vi "Tower_Crane_Balance_Monitor_beta.vi"() -> ()   [LabVIEW 2018]
uses:
  <vilib>/vision/driver/IMAQdx.llb/IMAQdx Acquisition Mode.ctl
  <vilib>/userdefined/High Color/IMAQdx.ctl
  <vilib>/Utility/error.llb/DialogType.ctl
  <vilib>/vision/driver/NI_Vision_Acquisition_Software.lvlib
panel:
  in  "File Path":path
  out "error out 2":errorcluster
  in  "error in":errorcluster
  in  "停止 3":bool
  out "视频监控画面1":T1(plugin-control)
  out "new picture 4":picture caption="Opertion_Guide"
  out "new picture 3":picture caption="Opertion_Guide"
  out "new picture 2":picture caption="Opertion_Guide"
  out "stanard_section 2":picture caption="配平状态"
  out "X倾斜角度 2":dbl caption="塔身X倾斜角度" format="%#_3g"
  out "Y倾斜角度  2":dbl caption="塔身Y倾斜角度" format="%#_3g"
  out "y轴倾角 2":dbl(knob) scale=0.0..5.0
  out "x轴倾角 2":dbl(knob) scale=0.0..5.0
  out "配平指示1":bool
  out "超声波雷达4":dbl format="%.3f"
  out "超声波雷达4 6":dbl(knob) scale=0.0..10.0
  out "超声波雷达35":dbl format="%.3f"
  out "?":dbl(knob) scale=0.0..10.0
  out "超声波雷达2":dbl format="%.3f"
  out "超声波雷达2":dbl(knob) scale=0.0..10.0
  out "超声波雷达1":dbl format="%.3f"
  out "超声波雷达1":dbl(knob) scale=0.0..10.0
  out "起升高度（m）":dbl caption="起升高度（cm）" format="%#_3g"
  out "变幅长度（m）":dbl format="%#_3g"
  out "风速（m/s）":dbl format="%.3f"
  out "Y倾斜角度":dbl caption="套架Y倾斜角度" format="%#_3g"
  out "X倾斜角度":dbl caption="套架X倾斜角度" format="%#_3g"
  out "回转角度（°）":dbl format="%#_3g"
  out "回转角度":dbl(knob) scale=0.0..10.0
  out "风速":dbl(knob) scale=0.0..10.0
  out "变幅长度":dbl(knob) scale=0.0..140.0
  out "y轴倾角":dbl(knob) scale=0.0..5.0
  out "x轴倾角":dbl(knob) scale=0.0..5.0
  out "起升高度":dbl(slide) caption="顶升高度          (cm)" scale=0.0..180.0
  out "section_connect":picture caption="引进节连接"
  out "rotary_support":picture caption="下回转支座"
  out "stanard_section":picture caption="引进节"
  out "pin_shaft":picture caption="爬爪"
  out "jacking_beam":picture caption="顶升横梁"
  out "new picture":picture caption="Opertion_Guide"
  out "引进滑轮":bool
  out "引进节螺栓4":bool
  out "引进节螺栓3":bool
  out "引进节螺栓2":bool
  out "引进节螺栓1":bool
  out "下回转螺栓4":bool
  out "下回转螺栓3":bool
  out "下回转螺栓2":bool
  out "下回转螺栓1":bool
  out "爬爪右侧":bool
  out "爬爪左侧":bool
  out "横梁右侧":bool
  out "横梁左侧":bool
  in  "倾角串口号 2":refnum<visa-resource-name>
  in  "开始配平":bool
  in  "倾角串口号":refnum<visa-resource-name>
  in  "风速串口号":refnum<visa-resource-name>
  in  "回转编码器":refnum<visa-resource-name>
  in  "变幅编码器":refnum<visa-resource-name>
  in  "高度编码器":refnum<visa-resource-name>
  in  "顶升开关":bool
  in  "滚轮直径D":dbl
  out "倾角读取缓冲区 2":string caption="倾角读取缓冲区"
  out "子字符串 4":string
  out "子字符串 3":string
  out "子字符串 2":string
  out "子字符串":string
  out "数据输出 2":string
  out "esp32的IP地址 2":string
  out "信息来源的端口 2":u16
  in  "清空 2":bool
  out "esp32的IP地址":string
  out "回转圈数":dbl
  out "回转编码器读取缓冲区":string
  out "回转单圈值":dbl
  out "回转编码器错误输出":string
  out "变幅圈数":dbl
  out "小车蝙蝠编码器读取缓冲区":string
  out "变幅单圈值":dbl
  out "回转编码器错误输出1":string
  out "倾角读取缓冲区":string
  out "Wind_Speed_Data":string
  out "风速传感器错误输出":string
  out "操作规范":string
  out "起升圈数":dbl
  out "起升高度编码器读取缓冲区 2":string
  out "起升单圈值":dbl
  out "起升高度编码器数值":dbl
  out "高度编码器错误输出1":string
  out "data out":string
  out "数据输出":string
  out "信息来源的端口":u16
  in  "停止":bool
  in  "清空":bool
types:
  T1 = typedef "IMAQ Image.ctl" = refnum<image>
  T2 = typedef "IMAQdx.ctl" = refnum<k21>
  T3 = typedef "NI_Vision_Acquisition_Software.lvlib/IMAQdx Acquisition Mode.ctl" = enum32{"One Shot", "Continuous"}
  T4 = typedef "DialogType.ctl" = u16
  T5 = typedef "imagedata.ctl" = cluster{"image type":i32, "image depth":i32, "image":u8[], "mask":u8[], "colors":u32[], "Rectangle":cluster{"left":i16, "top":i16, "right":i16, "bottom":i16}}
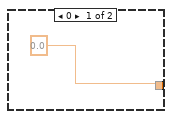
[diagram p2: hidden frame]
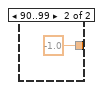
[diagram p4: hidden frame]
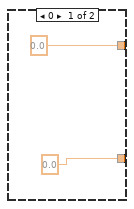
[diagram p9: hidden frame]
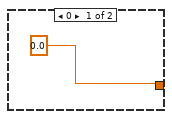
[diagram p14: hidden frame]
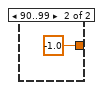
[diagram p16: hidden frame]
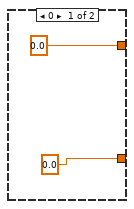
[diagram p17: hidden frame]
diagram:
  n1 = UDP Open(11:u16 8081 ("端口")) -> (port=w33:refnum<k16>, 0:w31:errorcluster)  [unwired: 4 in, 1 out]
  n2 = UDP Open(11:u16 8080 ("端口")) -> (port=w39:refnum<k16>, 0:w38:errorcluster)  [unwired: 4 in, 1 out]
  n3 = UDP Open(11:u16 8082 ("端口")) -> (port=w27:refnum<k16>, 0:w28:errorcluster)  [unwired: 4 in, 1 out]
  n4 = while {
    tunnel: w39 -> [w113]
    tunnel: w38 -> [w108]
    tunnel: [w141] -> w37
    tunnel: [w138] -> w36
    tunnel: w33 -> [w103]
    tunnel: [w101] -> w32
    tunnel: w31 -> [w99]
    tunnel: [w90] -> w30
    tunnel: w28 -> [w82]
    tunnel: w27 -> [w86]
    tunnel: [w81] -> w26
    tunnel: [w80] -> w25
    stop <- "停止" stop-if-true
    n5 = String To IP(1:"192.168.16.233" ("名称")) -> (0:w96:u32)
    n6 = String To IP(1:"192.168.16.236" ("名称")) -> (0:w110:u32)
    n7 = String To IP(1:"192.168.16.107" ("名称")) -> (0:w85:u32)
    n8 = UDP Write(address=w96, port or service name=u16 7780 ("端口或服务名称"), connection ID=w103, 8:w99) -> (error out=w100:errorcluster, 3:w102:refnum<k16>)  [unwired: 2 in]
    n9 = UDP Write(address=w110, port or service name=u16 7788 ("端口或服务名称"), connection ID=w113, 8:w108) -> (error out=w109:errorcluster, 3:w112:refnum<k16>)  [unwired: 2 in]
    n10 = Unbundle By Name(w82) -> ("code"=w83:i32)
    n11 = case shown="60" w83 {
      frame 0, Default {
      }
      frame 60 {
        n12 = Wait (ms)(milliseconds to wait=u32 5000 ("等待时间（毫秒）")) -> ()  [unwired: 1 out]
        n13 = One Button Dialog(message="目标端口被占用" ("消息"), button name ("OK")="难受" ("按钮名称（“确定”）")) -> ()  [unwired: 1 out]
      }
    }
    n14 = disable-structure shown="禁用" {
      disable-tunnel: [w142 _] -> w65
      frame Disabled {
        n15 = case shown="1, 默认" 1 {
          tunnel: [0.0 w150] -> w142
          frame 0 {
          }
          frame 1, Default {
            w148 = T4 0 items=["无对话框", "确定信息", "继续或停止信息", "确定信息＋警告", "继续/停止+警告"] ("type of dialog (OK msg:1)")
            w151 = i32[] [1, 3, 0, 2, 0, 2, 101, 203]  # 读指令
            n16 = Byte Array To String(unsigned byte array=w151) -> (string=w168:string)
            n17 = flat-sequence {
              tunnel: "变幅编码器" -> [w196]
              tunnel: [w196] -> w145
              frame #0 {
                n18 = Wait (ms)(milliseconds to wait=5) -> ()  [unwired: 1 out]
              }
            }
            n19 = flat-sequence {
              tunnel: [w194] -> w167
              tunnel: w168 -> [w194]
              frame #0 {
                n20 = Wait (ms)(milliseconds to wait=5) -> ()  [unwired: 1 out]
              }
            }
            n21 = VISA Write(VISA resource name=w145, write buffer=w167) -> (VISA resource name out=w159:refnum<visa-resource-name>)  [unwired: 1 in, 2 out]
            n22 = flat-sequence {
              tunnel: [w192] -> w160
              tunnel: w159 -> [w192]
              frame #0 {
                n23 = Wait (ms)(milliseconds to wait=5) -> ()  [unwired: 1 out]
              }
            }
            n24 = VISA Read(VISA resource name=w160, byte count=u32 9 ("字节总数")) -> (VISA resource name out=w176:refnum<visa-resource-name>, read buffer=w166:string, error out=w147:errorcluster)  [unwired: 1 in, 1 out]
            "小车蝙蝠编码器读取缓冲区" <- w166
            n25 = call <vilib>:"Simple Error Handler.vi"("type of dialog (OK msg:1)"=w148, "error in (no error)"=w147) -> ("error?"=w149:bool)  [unwired: 3 in, 4 out]
            n26 = case shown="真" w149 {
              frame False {
              }
              frame True {
                "回转编码器错误输出1" <- "小车变幅编码器丢失信号" ("九轴错误输出1")
              }
            }
            n27 = String To Byte Array(string=w166) -> (unsigned byte array=w174:u8[])
            n28 = VISA Flush I/O Buffer(VISA resource name=w176, mask (16)=64) -> (VISA resource name out=w175:refnum<visa-resource-name>)  [unwired: 1 in, 1 out]
            n29 = Index Array ("索引数组")(array=w174, index=3) -> (element=w161:u8)
            n30 = Index Array(array=w174, index=4) -> (element=w165:u8)
            n31 = Index Array ("索引数组")(array=w174, index=5) -> (element=w169:u8)
            n32 = Index Array(array=w174, index=6) -> (element=w173:u8)
            n33 = VISA Flush I/O Buffer(VISA resource name=w175, mask (16)=128) -> ()  [unwired: 1 in, 2 out]
            n34 = Number To Hexadecimal String(2:w161) -> (0:w164:string)  [unwired: 1 in]
            n35 = Number To Hexadecimal String(2:w165) -> (0:w163:string)  [unwired: 1 in]
            n36 = Number To Hexadecimal String(2:w169) -> (0:w172:string)  [unwired: 1 in]
            n37 = Number To Hexadecimal String(2:w173) -> (0:w171:string)  [unwired: 1 in]
            n38 = Concatenate Strings(w164, w163) -> (w162:string)
            n39 = Concatenate Strings(w172, w171) -> (w170:string)
            n40 = Hexadecimal String To Number(string=w162) -> (number=w177:u32)  [unwired: 2 in, 1 out]
            "变幅圈数" <- w177
            n41 = Hexadecimal String To Number(string=w170) -> (number=w178:u32)  [unwired: 2 in, 1 out]
            "变幅单圈值" <- w178
            n42 = case shown="默认" w177 {
              selector: w177 -> [w184 _]
              tunnel: w178 -> [w183 _]
              tunnel: [w182 -1.0] -> w150
              frame Default {
                n43 = Multiply(x=w184, y=1024.0) -> (x*y=w189:dbl)
                n44 = Add(x=w189, y=w183) -> (x+y=w190:dbl)
                n45 = Multiply(x=w190, y=0.001) -> (x*y=w187:dbl)
                n46 = Multiply(x=w187, y=3.141592653589793) -> (x*y=w188:dbl)
                n47 = Multiply(x=w188, y=3.0) -> (x*y=w182:dbl)
              }
              frame 90..99 {
              }
            }
          }
        }
      }
      frame Enabled {
      }
    }
    "变幅长度（m）" <- w65
    "变幅长度" <- w65
    n48 = Unbundle By Name(w108) -> ("code"=w132:i32)
    n49 = Unbundle By Name(w99) -> ("code"=w98:i32)
    n50 = case shown="60" w132 {
      frame 0, Default {
      }
      frame 60 {
        n51 = Wait (ms)(milliseconds to wait=u32 5000 ("等待时间（毫秒）")) -> ()  [unwired: 1 out]
        n52 = One Button Dialog(message="目标端口被占用" ("消息"), button name ("OK")="难受" ("按钮名称（“确定”）")) -> ()  [unwired: 1 out]
      }
    }
    n53 = case shown="60" w98 {
      frame 0, Default {
      }
      frame 60 {
        n54 = Wait (ms)(milliseconds to wait=u32 5000 ("等待时间（毫秒）")) -> ()  [unwired: 1 out]
        n55 = One Button Dialog(message="目标端口被占用" ("消息"), button name ("OK")="难受" ("按钮名称（“确定”）")) -> ()  [unwired: 1 out]
      }
    }
    n56 = case shown="1, 默认" 1 {
      tunnel: [0.0 w264] -> w64
      frame 0 {
      }
      frame 1, Default {
        w262 = T4 0 items=["无对话框", "确定信息", "继续或停止信息", "确定信息＋警告", "继续/停止+警告"] ("type of dialog (OK msg:1)")
        w265 = i32[] [1, 3, 0, 2, 0, 2, 101, 203]  # 读指令
        n57 = Byte Array To String(unsigned byte array=w265) -> (string=w282:string)
        n58 = flat-sequence {
          tunnel: "回转编码器" -> [w312]
          tunnel: [w312] -> w259
          frame #0 {
            n59 = Wait (ms)(milliseconds to wait=5) -> ()  [unwired: 1 out]
          }
        }
        n60 = flat-sequence {
          tunnel: [w310] -> w281
          tunnel: w282 -> [w310]
          frame #0 {
            n61 = Wait (ms)(milliseconds to wait=5) -> ()  [unwired: 1 out]
          }
        }
        n62 = VISA Write(VISA resource name=w259, write buffer=w281) -> (VISA resource name out=w273:refnum<visa-resource-name>)  [unwired: 1 in, 2 out]
        n63 = flat-sequence {
          tunnel: [w308] -> w274
          tunnel: w273 -> [w308]
          frame #0 {
            n64 = Wait (ms)(milliseconds to wait=5) -> ()  [unwired: 1 out]
          }
        }
        n65 = VISA Read(VISA resource name=w274, byte count=u32 9 ("字节总数")) -> (VISA resource name out=w290:refnum<visa-resource-name>, read buffer=w280:string, error out=w261:errorcluster)  [unwired: 1 in, 1 out]
        "回转编码器读取缓冲区" <- w280
        n66 = call <vilib>:"Simple Error Handler.vi"("type of dialog (OK msg:1)"=w262, "error in (no error)"=w261) -> ("error?"=w263:bool)  [unwired: 3 in, 4 out]
        n67 = case shown="真" w263 {
          frame False {
          }
          frame True {
            "回转编码器错误输出" <- "回转编码器丢失信号" ("九轴错误输出1")
          }
        }
        n68 = String To Byte Array(string=w280) -> (unsigned byte array=w288:u8[])
        n69 = VISA Flush I/O Buffer(VISA resource name=w290, mask (16)=64) -> (VISA resource name out=w289:refnum<visa-resource-name>)  [unwired: 1 in, 1 out]
        n70 = Index Array ("索引数组")(array=w288, index=3) -> (element=w275:u8)
        n71 = Index Array(array=w288, index=4) -> (element=w279:u8)
        n72 = Index Array ("索引数组")(array=w288, index=5) -> (element=w283:u8)
        n73 = Index Array(array=w288, index=6) -> (element=w287:u8)
        n74 = VISA Flush I/O Buffer(VISA resource name=w289, mask (16)=128) -> ()  [unwired: 1 in, 2 out]
        n75 = Number To Hexadecimal String(2:w275) -> (0:w278:string)  [unwired: 1 in]
        n76 = Number To Hexadecimal String(2:w279) -> (0:w277:string)  [unwired: 1 in]
        n77 = Number To Hexadecimal String(2:w283) -> (0:w286:string)  [unwired: 1 in]
        n78 = Number To Hexadecimal String(2:w287) -> (0:w285:string)  [unwired: 1 in]
        n79 = Concatenate Strings(w278, w277) -> (w276:string)
        n80 = Concatenate Strings(w286, w285) -> (w284:string)
        n81 = Hexadecimal String To Number(string=w276) -> (number=w291:u32)  [unwired: 2 in, 1 out]
        "回转圈数" <- w291
        n82 = Hexadecimal String To Number(string=w284) -> (number=w292:u32)  [unwired: 2 in, 1 out]
        "回转单圈值" <- w292
        n83 = case shown="默认" w291 {
          selector: w291 -> [w304 _]
          tunnel: w292 -> [w303 _]
          tunnel: [w295 -1.0] -> w264
          frame Default {
            n84 = Multiply(x=w304, y=1024.0) -> (x*y=w306:dbl)
            n85 = Add(x=w306, y=w303) -> (x+y=w302:dbl)
            n86 = Quotient & Remainder(x=w302, y=1024.0) -> (x-y*floor(x/y)=w297:dbl)  [unwired: 1 out]
            n87 = Divide(x=w297, y=1024.0) -> (x/y=w299:dbl)
            n88 = Multiply(x=w299, y=360.0) -> (x*y=w296:dbl)
            n89 = Divide(x=w296, y=10.0) -> (x/y=w295:dbl)
          }
          frame 90..99 {
          }
        }
      }
    }
    "回转角度（°）" <- w64
    "回转角度" <- w64
    n90 = disable-structure shown="禁用" {
      frame Disabled {
        n91 = case shown="1, 默认" 1 {
          tunnel: [0.0 w217] -> w211
          tunnel: [0.0 w223] -> w210
          frame 0 {
          }
          frame 1, Default {
            w220 = T4 0 items=["无对话框", "确定信息", "继续或停止信息", "确定信息＋警告", "继续/停止+警告"] ("type of dialog (OK msg:1)")
            w224 = i32[] [80, 3, 0, 61, 0, 3, 153, 134]  # 读指令
            # "javascript:placeObject(object906);"
            n92 = Byte Array To String(unsigned byte array=w224) -> (string=w236:string)
            n93 = flat-sequence {
              tunnel: "倾角串口号 2" -> [w256]
              tunnel: [w256] -> w218
              frame #0 {
                n94 = Wait (ms)(milliseconds to wait=5) -> ()  [unwired: 1 out]
              }
            }
            n95 = flat-sequence {
              tunnel: [w254] -> w215
              tunnel: w236 -> [w254]
              frame #0 {
                n96 = Wait (ms)(milliseconds to wait=5) -> ()  [unwired: 1 out]
              }
            }
            n97 = VISA Write(VISA resource name=w218, write buffer=w215) -> (VISA resource name out=w232:refnum<visa-resource-name>)  [unwired: 1 in, 2 out]
            n98 = flat-sequence {
              tunnel: w232 -> [w252]
              tunnel: [w252] -> w233
              frame #0 {
                n99 = Wait (ms)(milliseconds to wait=5) -> ()  [unwired: 1 out]
              }
            }
            n100 = VISA Read(VISA resource name=w233, byte count=u32 11 ("字节总数")) -> (VISA resource name out=w240:refnum<visa-resource-name>, read buffer=w216:string, error out=w221:errorcluster)  [unwired: 1 in, 1 out]
            "倾角读取缓冲区 2" <- w216
            n101 = call <vilib>:"Simple Error Handler.vi"("type of dialog (OK msg:1)"=w220, "error in (no error)"=w221) -> ("error?"=w222:bool)  [unwired: 3 in, 4 out]
            n102 = String To Byte Array(string=w216) -> (unsigned byte array=w241:u8[])
            n103 = VISA Flush I/O Buffer(VISA resource name=w240, mask (16)=64) -> (VISA resource name out=w239:refnum<visa-resource-name>)  [unwired: 1 in, 1 out]
            n104 = case shown="真" w222 {
              frame False {
              }
              frame True {
              }
            }
            n105 = Index Array(array=w241, index=5) -> (element=w238:u8)
            n106 = Index Array(array=w241, index=6) -> (element=w237:u8)
            n107 = Index Array(array=w241, index=3) -> (element=w235:u8)
            n108 = Index Array(array=w241, index=4) -> (element=w234:u8)
            n109 = formula code="z=((x<<8)|y)/32768*180;"("x"=w238, "y"=w237) -> ("z"=w243:dbl)
            n110 = formula code="z=((x<<8)|y)/32768*180;"("x"=w235, "y"=w234) -> ("z"=w242:dbl)
            n111 = VISA Flush I/O Buffer(VISA resource name=w239, mask (16)=128) -> ()  [unwired: 1 in, 2 out]
            n112 = case shown="300..360" w243 {
              tunnel: [w248 w250] -> w217
              tunnel: w243 -> [w248 w249]
              frame Default {
              }
              frame 300..360 {
                n113 = Subtract(x=360.0, y=w249) -> (x-y=w250:dbl)
              }
            }
            n114 = case shown="300..360" w242 {
              tunnel: [w244 w246] -> w223
              tunnel: w242 -> [w244 w245]
              frame Default {
              }
              frame 300..360 {
                n115 = Subtract(x=360.0, y=w245) -> (x-y=w246:dbl)
              }
            }
          }
        }
        "X倾斜角度 2" <- w210
        "Y倾斜角度  2" <- w211
        "y轴倾角 2" <- w211
        "x轴倾角 2" <- w210
        n116 = Number To Fractional String(number=w210) -> ()  [unwired: 3 in, 1 out]
        n117 = Number To Fractional String(number=w211) -> ()  [unwired: 3 in, 1 out]
      }
      frame Enabled {
      }
    }
    n118 = case shown="1, 默认" 1 {
      tunnel: [0.0 w400] -> w72
      frame 0 {
      }
      frame 1, Default {
        w398 = T4 0 items=["无对话框", "确定信息", "继续或停止信息", "确定信息＋警告", "继续/停止+警告"] ("type of dialog (OK msg:1)")
        w401 = i32[] [1, 3, 0, 2, 0, 2, 101, 203]  # 读指令
        n119 = Byte Array To String(unsigned byte array=w401) -> (string=w417:string)
        n120 = flat-sequence {
          tunnel: "高度编码器" -> [w446]
          tunnel: [w446] -> w395
          frame #0 {
            n121 = Wait (ms)(milliseconds to wait=5) -> ()  [unwired: 1 out]
          }
        }
        n122 = flat-sequence {
          tunnel: [w444] -> w416
          tunnel: w417 -> [w444]
          frame #0 {
            n123 = Wait (ms)(milliseconds to wait=5) -> ()  [unwired: 1 out]
          }
        }
        n124 = VISA Write(VISA resource name=w395, write buffer=w416) -> (VISA resource name out=w409:refnum<visa-resource-name>)  [unwired: 1 in, 2 out]
        n125 = flat-sequence {
          tunnel: [w442] -> w410
          tunnel: w409 -> [w442]
          frame #0 {
            n126 = Wait (ms)(milliseconds to wait=5) -> ()  [unwired: 1 out]
          }
        }
        n127 = VISA Read(VISA resource name=w410, byte count=u32 9 ("字节总数")) -> (VISA resource name out=w425:refnum<visa-resource-name>, read buffer=w426:string, error out=w397:errorcluster)  [unwired: 1 in, 1 out]
        "起升高度编码器读取缓冲区 2" <- w426
        n128 = call <vilib>:"Simple Error Handler.vi"("type of dialog (OK msg:1)"=w398, "error in (no error)"=w397) -> ("error?"=w399:bool)  [unwired: 3 in, 4 out]
        n129 = case shown="假" w399 {
          frame False {
          }
          frame True {
            "高度编码器错误输出1" <- "起升高度编码器丢失信号" ("九轴错误输出1")
          }
        }
        n130 = String To Byte Array(string=w426) -> (unsigned byte array=w423:u8[])
        n131 = VISA Flush I/O Buffer(VISA resource name=w425, mask (16)=64) -> (VISA resource name out=w424:refnum<visa-resource-name>)  [unwired: 1 in, 1 out]
        n132 = Index Array ("索引数组")(array=w423, index=3) -> (element=w411:u8)
        n133 = Index Array(array=w423, index=4) -> (element=w415:u8)
        n134 = Index Array ("索引数组")(array=w423, index=5) -> (element=w418:u8)
        n135 = Index Array(array=w423, index=6) -> (element=w422:u8)
        n136 = VISA Flush I/O Buffer(VISA resource name=w424, mask (16)=128) -> ()  [unwired: 1 in, 2 out]
        n137 = Number To Hexadecimal String(2:w411) -> (0:w414:string)  [unwired: 1 in]
        n138 = Number To Hexadecimal String(2:w415) -> (0:w413:string)  [unwired: 1 in]
        n139 = Number To Hexadecimal String(2:w418) -> (0:w421:string)  [unwired: 1 in]
        n140 = Number To Hexadecimal String(2:w422) -> (0:w420:string)  [unwired: 1 in]
        n141 = Concatenate Strings(w414, w413) -> (w412:string)
        n142 = Concatenate Strings(w421, w420) -> (w419:string)
        n143 = Hexadecimal String To Number(string=w412) -> (number=w427:u32)  [unwired: 2 in, 1 out]
        "起升圈数" <- w427
        n144 = Hexadecimal String To Number(string=w419) -> (number=w428:u32)  [unwired: 2 in, 1 out]
        "起升单圈值" <- w428
        n145 = case shown="默认" w427 {
          selector: w427 -> [w437 _]
          tunnel: w428 -> [w438 _]
          tunnel: [w430 -1.0] -> w400
          frame Default {
            n146 = Multiply(x=w437, y=1024.0) -> (x*y=w440:dbl)
            n147 = Add(x=w440, y=w438) -> (x+y=w436:dbl)
            "起升高度编码器数值" <- w436
            n148 = Divide(x=w436, y=1024.0) -> (x/y=w434:dbl)
            n149 = Multiply(x=w434, y=3.141592653589793) -> (x*y=w432:dbl)
            n150 = Multiply(x=w432, y="滚轮直径D") -> (x*y=w430:dbl)
          }
          frame 90..99 {
          }
        }
      }
    }
    "起升高度（m）" <- w72
    "起升高度" <- w72
    n151 = case shown="1, 默认" 1 {
      tunnel: [0.0 w322] -> w48
      tunnel: [0.0 w321] -> w46
      frame 0 {
      }
      frame 1, Default {
        w318 = T4 0 items=["无对话框", "确定信息", "继续或停止信息", "确定信息＋警告", "继续/停止+警告"] ("type of dialog (OK msg:1)")
        w323 = i32[] [80, 3, 0, 61, 0, 3, 153, 134]  # 读指令
        # "javascript:placeObject(object906);"
        n152 = Byte Array To String(unsigned byte array=w323) -> (string=w336:string)
        n153 = flat-sequence {
          tunnel: [w357] -> w317
          tunnel: "倾角串口号" -> [w357]
          frame #0 {
            n154 = Wait (ms)(milliseconds to wait=5) -> ()  [unwired: 1 out]
          }
        }
        n155 = flat-sequence {
          tunnel: [w355] -> w337
          tunnel: w336 -> [w355]
          frame #0 {
            n156 = Wait (ms)(milliseconds to wait=5) -> ()  [unwired: 1 out]
          }
        }
        n157 = VISA Write(VISA resource name=w317, write buffer=w337) -> (VISA resource name out=w332:refnum<visa-resource-name>)  [unwired: 1 in, 2 out]
        n158 = flat-sequence {
          tunnel: w332 -> [w353]
          tunnel: [w353] -> w333
          frame #0 {
            n159 = Wait (ms)(milliseconds to wait=5) -> ()  [unwired: 1 out]
          }
        }
        n160 = VISA Read(VISA resource name=w333, byte count=u32 11 ("字节总数")) -> (VISA resource name out=w341:refnum<visa-resource-name>, read buffer=w331:string, error out=w319:errorcluster)  [unwired: 1 in, 1 out]
        "倾角读取缓冲区" <- w331
        n161 = call <vilib>:"Simple Error Handler.vi"("type of dialog (OK msg:1)"=w318, "error in (no error)"=w319) -> ("error?"=w320:bool)  [unwired: 3 in, 4 out]
        n162 = String To Byte Array(string=w331) -> (unsigned byte array=w342:u8[])
        n163 = VISA Flush I/O Buffer(VISA resource name=w341, mask (16)=64) -> (VISA resource name out=w340:refnum<visa-resource-name>)  [unwired: 1 in, 1 out]
        n164 = case shown="真" w320 {
          frame False {
          }
          frame True {
          }
        }
        n165 = Index Array(array=w342, index=5) -> (element=w339:u8)
        n166 = Index Array(array=w342, index=6) -> (element=w338:u8)
        n167 = Index Array(array=w342, index=3) -> (element=w335:u8)
        n168 = Index Array(array=w342, index=4) -> (element=w334:u8)
        n169 = formula code="z=((x<<8)|y)/32768*180;"("x"=w339, "y"=w338) -> ("z"=w344:dbl)
        n170 = formula code="z=((x<<8)|y)/32768*180;"("x"=w335, "y"=w334) -> ("z"=w343:dbl)
        n171 = VISA Flush I/O Buffer(VISA resource name=w340, mask (16)=128) -> ()  [unwired: 1 in, 2 out]
        n172 = case shown="300..360" w344 {
          tunnel: [w349 w351] -> w322
          tunnel: w344 -> [w349 w350]
          frame Default {
          }
          frame 300..360 {
            n173 = Subtract(x=360.0, y=w350) -> (x-y=w351:dbl)
          }
        }
        n174 = case shown="300..360" w343 {
          tunnel: [w345 w347] -> w321
          tunnel: w343 -> [w345 w346]
          frame Default {
          }
          frame 300..360 {
            n175 = Subtract(x=360.0, y=w346) -> (x-y=w347:dbl)
          }
        }
      }
    }
    "X倾斜角度" <- w46
    "Y倾斜角度" <- w48
    "x轴倾角" <- w48
    "y轴倾角" <- w46
    n176 = case shown="1, 默认" 1 {
      tunnel: [u32 0 w361] -> w42
      frame 0 {
      }
      frame 1, Default {
        w375 = T4 0 items=["无对话框", "确定信息", "继续或停止信息", "确定信息＋警告", "继续/停止+警告"] ("type of dialog (OK msg:1)")
        w377 = i32[] [1, 3, 0, 0, 0, 1, 132, 10]  # 读指令
        n177 = Byte Array To String(unsigned byte array=w377) -> (string=w384:string)
        n178 = flat-sequence {
          tunnel: "风速串口号" -> [w392]
          tunnel: [w392] -> w372
          frame #0 {
            n179 = Wait (ms)(milliseconds to wait=5) -> ()  [unwired: 1 out]
          }
        }
        n180 = flat-sequence {
          tunnel: [w390] -> w383
          tunnel: w384 -> [w390]
          frame #0 {
            n181 = Wait (ms)(milliseconds to wait=5) -> ()  [unwired: 1 out]
          }
        }
        n182 = VISA Write(VISA resource name=w372, write buffer=w383) -> (VISA resource name out=w381:refnum<visa-resource-name>)  [unwired: 1 in, 2 out]
        n183 = flat-sequence {
          tunnel: [w388] -> w382
          tunnel: w381 -> [w388]
          frame #0 {
            n184 = Wait (ms)(milliseconds to wait=5) -> ()  [unwired: 1 out]
          }
        }
        n185 = VISA Read(VISA resource name=w382, byte count=u32 7 ("字节总数")) -> (VISA resource name out=w386:refnum<visa-resource-name>, read buffer=w371:string, error out=w374:errorcluster)  [unwired: 1 in, 1 out]
        "Wind_Speed_Data" <- w371
        n186 = call <vilib>:"Simple Error Handler.vi"("type of dialog (OK msg:1)"=w375, "error in (no error)"=w374) -> ("error?"=w376:bool)  [unwired: 3 in, 4 out]
        n187 = case shown="真" w376 {
          frame False {
          }
          frame True {
            "风速传感器错误输出" <- "Wnd_Sensor_Signal_Loss" ("九轴错误输出1")
          }
        }
        n188 = VISA Flush I/O Buffer(VISA resource name=w386, mask (16)=64) -> (VISA resource name out=w385:refnum<visa-resource-name>)  [unwired: 1 in, 1 out]
        n189 = VISA Flush I/O Buffer(VISA resource name=w385, mask (16)=128) -> ()  [unwired: 1 in, 2 out]
        n190 = String To Byte Array(string=w371) -> (unsigned byte array=w370:u8[])
        n191 = Index Array(array=w370, index=3 ("索引")) -> (element=w367:u8)
        n192 = Index Array(array=w370, index=4 ("索引")) -> (element=w366:u8)
        n193 = Number To Hexadecimal String(2:w367) -> (0:w365:string)  [unwired: 1 in]
        n194 = Number To Hexadecimal String(2:w366) -> (0:w364:string)  [unwired: 1 in]
        n195 = Concatenate Strings(w365, w364) -> (w363:string)
        n196 = Hexadecimal String To Number(string=w363) -> (number=w362:u32)  [unwired: 2 in, 1 out]
        n197 = Multiply(x=w362, y=0.1) -> (x*y=w361:dbl)
      }
    }
    "风速" <- w42
    "风速（m/s）" <- w42
    n198 = UDP Read(connection ID=w112, max size (548)=548 ("最大值(548)"), timeout ms (25000)=10 ("超时毫秒(25000)"), 8:w109) -> (data out=w55:string, error out=w141:errorcluster, 3:w138:refnum<k16>, 4:w131:u16, 6:w135:u32)
    n199 = String Length(string=w55) -> (length=w137:i32)
    n200 = UDP Read(connection ID=w102, max size (548)=548 ("最大值(548)"), timeout ms (25000)=10 ("超时毫秒(25000)"), 8:w100) -> (data out=w54:string, error out=w90:errorcluster, 3:w101:refnum<k16>, 4:w91:u16, 6:w92:u32)
    n201 = Not Equal To 0?(x=w131) -> (x != 0?=w133:bool)
    n202 = Not Equal To 0?(x=w135) -> (x != 0?=w134:bool)
    n203 = Not Equal To 0?(x=w92) -> (x != 0?=w104:bool)
    n204 = Not Equal To 0?(x=w91) -> (x != 0?=w105:bool)
    n205 = Not Equal To 0?(x=w137) -> (x != 0?=w136:bool)
    n206 = case shown="真" w134 {
      tunnel: w135 -> [_ w501]
      frame False {
      }
      frame True {
        n207 = IP To String(1:TRUE ("句点符号？(F)"), 2:w501) -> (0:→"esp32的IP地址":string)
      }
    }
    n208 = case shown="真" w104 {
      tunnel: w92 -> [_ w491]
      frame False {
      }
      frame True {
        n209 = IP To String(1:TRUE ("句点符号？(F)"), 2:w491) -> (0:→"esp32的IP地址 2":string)
      }
    }
    n210 = case shown="真" w133 {
      tunnel: w131 -> [_ w498]
      frame False {
      }
      frame True {
        "信息来源的端口" <- w498
      }
    }
    n211 = case shown="真" w105 {
      tunnel: w91 -> [_ w490]
      frame False {
      }
      frame True {
        "信息来源的端口 2" <- w490
      }
    }
    n212 = case shown="真" w136 {
      tunnel: w55 -> [_ w505]
      tunnel: w72 -> [_ w503]
      frame False {
      }
      frame True {
        n213 = local read "顶升开关"() -> (w502:bool)
        n214 = local read "数据输出"() -> (w506:string)
        n215 = case shown="真" w502 {
          tunnel: w506 -> [w509 w618]
          tunnel: w505 -> [w508 w593]
          tunnel: w503 -> [_ w596]
          frame False {
            n216 = Concatenate Strings(w509, w508) -> (w507:string)
            n217 = local write "数据输出"(w507) -> ()
          }
          frame True {
            (unwired) 0 ("默认(0 I32)")
            n218 = Concatenate Strings(w618, "\n", w593) -> (→"数据输出":string)
            n219 = String Subset(string=w593, offset (0)=22 ("偏移量(0)"), length (rest)=1 ("长度（剩余）")) -> (substring=w554:string)
            n220 = String Subset(string=w593, offset (0)=25 ("偏移量(0)"), length (rest)=1 ("长度（剩余）")) -> (substring=w553:string)
            n221 = String Subset(string=w593, offset (0)=19 ("偏移量(0)"), length (rest)=1 ("长度（剩余）")) -> (substring=w555:string)
            n222 = String Subset(string=w593, offset (0)=28 ("偏移量(0)"), length (rest)=1 ("长度（剩余）")) -> (substring=w552:string)
            n223 = String Subset(string=w593, offset (0)=37 ("偏移量(0)"), length (rest)=1 ("长度（剩余）")) -> (substring=w549:string)
            n224 = String Subset(string=w593, offset (0)=16 ("偏移量(0)"), length (rest)=1 ("长度（剩余）")) -> (substring=w571:string)
            n225 = String Subset(string=w593, offset (0)=4 ("偏移量(0)"), length (rest)=1 ("长度（剩余）")) -> (substring=w606:string)
            n226 = String Subset(string=w593, offset (0)=13 ("偏移量(0)"), length (rest)=1 ("长度（剩余）")) -> (substring=w572:string)
            n227 = String Subset(string=w593, offset (0)=1 ("偏移量(0)"), length (rest)=1 ("长度（剩余）")) -> (substring=w608:string)
            n228 = String Subset(string=w593, offset (0)=10 ("偏移量(0)"), length (rest)=1 ("长度（剩余）")) -> (substring=w605:string)
            n229 = String Subset(string=w593, offset (0)=31 ("偏移量(0)"), length (rest)=1 ("长度（剩余）")) -> (substring=w551:string)
            n230 = String Subset(string=w593, offset (0)=7 ("偏移量(0)"), length (rest)=1 ("长度（剩余）")) -> (substring=w607:string)
            n231 = String Subset(string=w593, offset (0)=34 ("偏移量(0)"), length (rest)=1 ("长度（剩余）")) -> (substring=w550:string)
            n232 = Decimal String To Number(string=w555, offset=0 ("偏移量"), default (0L)=0 ("默认(0 I32)")) -> (number=w525:i32)  [unwired: 1 out]
            n233 = Decimal String To Number(string=w606, offset=0 ("偏移量"), default (0L)=0 ("默认(0 I32)")) -> (number=w533:i32)  [unwired: 1 out]
            n234 = Decimal String To Number(string=w554, offset=0 ("偏移量"), default (0L)=0 ("默认(0 I32)")) -> (number=w524:i32)  [unwired: 1 out]
            n235 = Decimal String To Number(string=w607, offset=0 ("偏移量"), default (0L)=0 ("默认(0 I32)")) -> (number=w531:i32)  [unwired: 1 out]
            n236 = Decimal String To Number(string=w572, offset=0 ("偏移量"), default (0L)=0 ("默认(0 I32)")) -> (number=w527:i32)  [unwired: 1 out]
            n237 = Decimal String To Number(string=w553, offset=0 ("偏移量")) -> (number=w523:i32)  [unwired: 1 in, 1 out]
            n238 = Decimal String To Number(string=w571, offset=0 ("偏移量"), default (0L)=0 ("默认(0 I32)")) -> (number=w526:i32)  [unwired: 1 out]
            n239 = Decimal String To Number(string=w605, offset=0 ("偏移量"), default (0L)=0 ("默认(0 I32)")) -> (number=w529:i32)  [unwired: 1 out]
            n240 = Decimal String To Number(string=w608, offset=0 ("偏移量"), default (0L)=0 ("默认(0 I32)")) -> (number=w548:i32)  [unwired: 1 out]
            n241 = Decimal String To Number(string=w552, offset=0 ("偏移量"), default (0L)=0 ("默认(0 I32)")) -> (number=w522:i32)  [unwired: 1 out]
            n242 = Decimal String To Number(string=w551, offset=0 ("偏移量"), default (0L)=0 ("默认(0 I32)")) -> (number=w521:i32)  [unwired: 1 out]
            n243 = Decimal String To Number(string=w550, offset=0 ("偏移量"), default (0L)=0 ("默认(0 I32)")) -> (number=w520:i32)  [unwired: 1 out]
            n244 = Decimal String To Number(string=w549, offset=0 ("偏移量"), default (0L)=0 ("默认(0 I32)")) -> (number=w519:i32)  [unwired: 1 out]
            n245 = Equal?(x=w533, y=1) -> (x = y?=→"横梁右侧":bool)
            n246 = Equal?(x=w548, y=1) -> (x = y?=→"横梁左侧":bool)
            n247 = Equal?(x=w520, y=1) -> (x = y?=→"引进节螺栓4":bool)
            n248 = Equal?(x=w521, y=1) -> (x = y?=→"引进节螺栓3":bool)
            n249 = Equal?(x=w526, y=1) -> (x = y?=→"下回转螺栓2":bool)
            n250 = Equal?(x=w525, y=1) -> (x = y?=→"下回转螺栓3":bool)
            n251 = Equal?(x=w524, y=1) -> (x = y?=→"下回转螺栓4":bool)
            n252 = Equal?(x=w527, y=1) -> (x = y?=→"下回转螺栓1":bool)
            n253 = Equal?(x=w519, y=1) -> (x = y?=→"引进滑轮":bool)
            n254 = Equal?(x=w529, y=1) -> (x = y?=→"爬爪右侧":bool)
            n255 = Equal?(x=w531, y=1) -> (x = y?=→"爬爪左侧":bool)
            n256 = To Word Integer(number=w596) -> (16bit integer=w595:i16)
            n257 = Equal?(x=w522, y=1) -> (x = y?=→"引进节螺栓2":bool)
            n258 = Equal?(x=w523, y=1) -> (x = y?=→"引进节螺栓1":bool)
            n259 = case shown="50..60" w595 {
              tunnel: w548 -> [w634 w749 w964 w1042 w1117 _ w1199]
              tunnel: w533 -> [w633 w748 w965 w1041 w1116 _ w1198]
              tunnel: w531 -> [w632 w747 w963 w1040 w1115 _ w1197]
              tunnel: w529 -> [w631 w746 w962 w1039 w1114 _ w1196]
              tunnel: w527 -> [w630 w745 w961 w1038 w1113 _ w1195]
              tunnel: w526 -> [w629 w744 w960 w1037 w1112 _ w1194]
              tunnel: w525 -> [w628 w743 w959 w1036 w1111 _ w1193]
              tunnel: w524 -> [w627 w742 w958 w1035 w1110 _ w1192]
              tunnel: w523 -> [w626 w741 w957 w1034 w1109 _ w1191]
              tunnel: w522 -> [w625 w734 w956 w1033 w1108 _ w1190]
              tunnel: w521 -> [w624 w740 w955 w1032 w1107 _ w1189]
              tunnel: w520 -> [w623 w739 w954 w1031 w1106 _ w1188]
              tunnel: w519 -> [w622 w738 w953 w1030 w1105 _ w1187]
              frame 25..30, Default {
                n260 = Equal?(x=w634, y=0) -> (x = y?=w712:bool)
                n261 = Equal?(x=w633, y=0) -> (x = y?=w711:bool)
                n262 = Equal?(x=w623, y=0) -> (x = y?=w701:bool)
                n263 = Equal?(x=w622, y=0) -> (x = y?=w700:bool)
                n264 = Equal?(x=w624, y=0) -> (x = y?=w702:bool)
                n265 = Equal?(x=w626, y=0) -> (x = y?=w704:bool)
                n266 = Equal?(x=w632, y=1) -> (x = y?=w710:bool)
                n267 = Equal?(x=w627, y=0) -> (x = y?=w705:bool)
                n268 = Equal?(x=w629, y=0) -> (x = y?=w707:bool)
                n269 = Equal?(x=w630, y=0) -> (x = y?=w708:bool)
                n270 = Equal?(x=w628, y=0) -> (x = y?=w706:bool)
                n271 = Equal?(x=w625, y=0) -> (x = y?=w703:bool)
                n272 = Equal?(x=w631, y=1) -> (x = y?=w709:bool)
                n273 = Compound Arithmetic op=AND ("复合运算")(w712, w711, w710, w709, w708, w707, w706, w705, w704, w703, w702, w701, w700) -> (w621:bool)
                n274 = Equal?(x=w634, y=1) -> (x = y?=w687:bool)
                n275 = Equal?(x=w633, y=1) -> (x = y?=w688:bool)
                n276 = Equal?(x=w623, y=0) -> (x = y?=w698:bool)
                n277 = Equal?(x=w622, y=0) -> (x = y?=w699:bool)
                n278 = Equal?(x=w624, y=0) -> (x = y?=w697:bool)
                n279 = Equal?(x=w626, y=0) -> (x = y?=w695:bool)
                n280 = Equal?(x=w632, y=1) -> (x = y?=w689:bool)
                n281 = Equal?(x=w627, y=0) -> (x = y?=w694:bool)
                n282 = Equal?(x=w629, y=0) -> (x = y?=w692:bool)
                n283 = Equal?(x=w630, y=0) -> (x = y?=w691:bool)
                n284 = Equal?(x=w628, y=0) -> (x = y?=w693:bool)
                n285 = Equal?(x=w625, y=0) -> (x = y?=w696:bool)
                n286 = Equal?(x=w631, y=1) -> (x = y?=w690:bool)
                n287 = Compound Arithmetic op=AND ("复合运算")(w687, w688, w689, w690, w691, w692, w693, w694, w695, w696, w697, w698, w699) -> (w620:bool)
                n288 = Equal?(x=w634, y=1) -> (x = y?=w686:bool)
                n289 = Equal?(x=w633, y=1) -> (x = y?=w685:bool)
                n290 = Equal?(x=w623, y=0) -> (x = y?=w675:bool)
                n291 = Equal?(x=w622, y=0) -> (x = y?=w674:bool)
                n292 = Equal?(x=w624, y=0) -> (x = y?=w676:bool)
                n293 = Equal?(x=w626, y=0) -> (x = y?=w678:bool)
                n294 = Equal?(x=w632, y=0) -> (x = y?=w684:bool)
                n295 = Equal?(x=w627, y=0) -> (x = y?=w679:bool)
                n296 = Equal?(x=w629, y=0) -> (x = y?=w681:bool)
                n297 = Equal?(x=w630, y=0) -> (x = y?=w682:bool)
                n298 = Equal?(x=w628, y=0) -> (x = y?=w680:bool)
                n299 = Equal?(x=w625, y=0) -> (x = y?=w677:bool)
                n300 = Equal?(x=w631, y=0) -> (x = y?=w683:bool)
                n301 = Compound Arithmetic op=AND ("复合运算")(w686, w685, w684, w683, w682, w681, w680, w679, w678, w677, w676, w675, w674) -> (w619:bool)
                n302 = case shown="真" w620 {
                  frame False {
                    n303 = call "Empty Picture"() -> ("empty picture"=w714:picture)
                    n304 = local write "new picture"(w714) -> ()
                    n305 = local write "操作规范"("" ("字符串")) -> ()
                  }
                  frame True {
                    n306 = call <vilib>:"Read PNG File.vi"("path to PNG file"=path "Picture_Data/1.png" ("path to JPEG file")) -> ("image data"=w719:T5)  [unwired: 8 in, 2 out]
                    n307 = call <vilib>:"Draw Flattened Pixmap.vi"("image data"=w719) -> ("new picture"=w715:picture)  [unwired: 8 in]
                    n308 = One Button Dialog(message="顶升横梁与踏步连接销轴已连接，请掀起爬爪！" ("消息")) -> ()  [unwired: 1 in, 1 out]
                    n309 = local write "操作规范"("顶升横梁与踏步连接销轴已连接，请掀起爬爪！" ("字符串")) -> ()
                    n310 = local write "new picture"(w715) -> ()
                  }
                }
                n311 = case shown="真" w621 {
                  frame False {
                    n312 = call "Empty Picture"() -> ("empty picture"=w727:picture)
                    n313 = local write "new picture"(w727) -> ()
                    n314 = local write "操作规范"("" ("字符串")) -> ()
                  }
                  frame True {
                    n315 = call <vilib>:"Read PNG File.vi"("path to PNG file"=path "Picture_Data/1.png" ("path to JPEG file")) -> ("image data"=w733:T5)  [unwired: 8 in, 2 out]
                    n316 = call <vilib>:"Draw Flattened Pixmap.vi"("image data"=w733) -> ("new picture"=w729:picture)  [unwired: 8 in]
                    n317 = One Button Dialog(message="油缸压缩完毕，请连接顶升横梁与踏步连接销轴！" ("消息")) -> ()  [unwired: 1 in, 1 out]
                    n318 = local write "操作规范"("油缸压缩完毕，请连接顶升横梁与踏步连接销轴！" ("字符串")) -> ()
                    n319 = local write "new picture"(w729) -> ()
                  }
                }
                n320 = case shown="真" w619 {
                  frame False {
                    n321 = call "Empty Picture"() -> ("empty picture"=w720:picture)
                    n322 = local write "new picture"(w720) -> ()
                    n323 = local write "操作规范"("" ("字符串")) -> ()
                  }
                  frame True {
                    n324 = call <vilib>:"Read PNG File.vi"("path to PNG file"=path "Picture_Data/1.png" ("path to JPEG file")) -> ("image data"=w726:T5)  [unwired: 8 in, 2 out]
                    n325 = call <vilib>:"Draw Flattened Pixmap.vi"("image data"=w726) -> ("new picture"=w723:picture)  [unwired: 8 in]
                    n326 = local write "操作规范"("爬爪已掀起，请出缸顶升至容纳引进节！" ("字符串")) -> ()
                    n327 = One Button Dialog(message="爬爪已掀起，请出缸顶升至容纳引进节！" ("消息")) -> ()  [unwired: 1 in, 1 out]
                    n328 = local write "new picture"(w723) -> ()
                  }
                }
              }
              frame 50..60 {
                n329 = Equal?(x=w749, y=0) -> (x = y?=w908:bool)
                n330 = Equal?(x=w748, y=0) -> (x = y?=w907:bool)
                n331 = Equal?(x=w739, y=0) -> (x = y?=w897:bool)
                n332 = Equal?(x=w738, y=0) -> (x = y?=w896:bool)
                n333 = Equal?(x=w740, y=0) -> (x = y?=w898:bool)
                n334 = Equal?(x=w741, y=0) -> (x = y?=w900:bool)
                n335 = Equal?(x=w747, y=0) -> (x = y?=w906:bool)
                n336 = Equal?(x=w742, y=1) -> (x = y?=w901:bool)
                n337 = Equal?(x=w744, y=1) -> (x = y?=w903:bool)
                n338 = Equal?(x=w745, y=1) -> (x = y?=w904:bool)
                n339 = Equal?(x=w743, y=1) -> (x = y?=w902:bool)
                n340 = Equal?(x=w734, y=0) -> (x = y?=w899:bool)
                n341 = Equal?(x=w746, y=0) -> (x = y?=w905:bool)
                n342 = Compound Arithmetic op=AND ("复合运算")(w908, w907, w906, w905, w904, w903, w902, w901, w900, w899, w898, w897, w896) -> (w830:bool)
                n343 = case shown="真" w830 {
                  frame False {
                    n344 = call "Empty Picture"() -> ("empty picture"=w945:picture)
                    n345 = local write "new picture"(w945) -> ()
                    n346 = local write "操作规范"("" ("字符串")) -> ()
                  }
                  frame True {
                    n347 = call <vilib>:"Read PNG File.vi"("path to PNG file"=path "Picture_Data/1.png" ("path to JPEG file")) -> ("image data"=w949:T5)  [unwired: 8 in, 2 out]
                    n348 = call <vilib>:"Draw Flattened Pixmap.vi"("image data"=w949) -> ("new picture"=→"new picture":picture)  [unwired: 8 in]
                    n349 = One Button Dialog(message="顶升作业开始，请操作顶升油缸伸长并连接顶升横梁与踏步！" ("消息")) -> ()  [unwired: 1 in, 1 out]
                    "操作规范" <- "顶升作业开始，请操作顶升油缸伸长并连接顶升横梁与踏步！" ("字符串")
                  }
                }
                n350 = Equal?(x=w749, y=1) -> (x = y?=w883:bool)
                n351 = Equal?(x=w748, y=1) -> (x = y?=w884:bool)
                n352 = Equal?(x=w739, y=0) -> (x = y?=w894:bool)
                n353 = Equal?(x=w738, y=0) -> (x = y?=w895:bool)
                n354 = Equal?(x=w740, y=0) -> (x = y?=w893:bool)
                n355 = Equal?(x=w741, y=0) -> (x = y?=w891:bool)
                n356 = Equal?(x=w747, y=0) -> (x = y?=w885:bool)
                n357 = Equal?(x=w742, y=1) -> (x = y?=w890:bool)
                n358 = Equal?(x=w744, y=1) -> (x = y?=w888:bool)
                n359 = Equal?(x=w745, y=1) -> (x = y?=w887:bool)
                n360 = Equal?(x=w743, y=1) -> (x = y?=w889:bool)
                n361 = Equal?(x=w734, y=0) -> (x = y?=w892:bool)
                n362 = Equal?(x=w746, y=0) -> (x = y?=w886:bool)
                n363 = Compound Arithmetic op=AND ("复合运算")(w883, w884, w885, w886, w887, w888, w889, w890, w891, w892, w893, w894, w895) -> (w750:bool)
                n364 = Equal?(x=w749, y=1) -> (x = y?=w882:bool)
                n365 = Equal?(x=w748, y=1) -> (x = y?=w881:bool)
                n366 = Equal?(x=w739, y=0) -> (x = y?=w871:bool)
                n367 = Equal?(x=w738, y=0) -> (x = y?=w870:bool)
                n368 = Equal?(x=w740, y=0) -> (x = y?=w872:bool)
                n369 = Equal?(x=w741, y=0) -> (x = y?=w874:bool)
                n370 = Equal?(x=w747, y=0) -> (x = y?=w880:bool)
                n371 = Equal?(x=w742, y=0) -> (x = y?=w875:bool)
                n372 = Equal?(x=w744, y=0) -> (x = y?=w877:bool)
                n373 = Equal?(x=w745, y=0) -> (x = y?=w878:bool)
                n374 = Equal?(x=w743, y=0) -> (x = y?=w876:bool)
                n375 = Equal?(x=w734, y=0) -> (x = y?=w873:bool)
                n376 = Equal?(x=w746, y=0) -> (x = y?=w879:bool)
                n377 = Compound Arithmetic op=AND ("复合运算")(w882, w881, w880, w879, w878, w877, w876, w875, w874, w873, w872, w871, w870) -> (w829:bool)
                n378 = case shown="真" w829 {
                  frame False {
                    n379 = call "Empty Picture"() -> ("empty picture"=w931:picture)
                    n380 = local write "new picture"(w931) -> ()
                    n381 = local write "操作规范"("" ("字符串")) -> ()
                  }
                  frame True {
                    n382 = call <vilib>:"Read PNG File.vi"("path to PNG file"=path "C:/Users/Dr.Pei/Desktop/1.png" ("path to JPEG file")) -> ("image data"=w935:T5)  [unwired: 8 in, 2 out]
                    n383 = One Button Dialog(message="下回转与塔身连接已取消，请出缸顶升！" ("消息")) -> ()  [unwired: 1 in, 1 out]
                    n384 = call <vilib>:"Draw Flattened Pixmap.vi"("image data"=w935) -> ("new picture"=w934:picture)  [unwired: 8 in]
                    n385 = local write "操作规范"("下回转与塔身连接已取消，请出缸顶升！" ("字符串")) -> ()
                    n386 = local write "new picture"(w934) -> ()
                  }
                }
                n387 = case shown="真" w750 {
                  frame False {
                    n388 = call "Empty Picture"() -> ("empty picture"=w938:picture)
                    n389 = local write "操作规范"("" ("字符串")) -> ()
                    n390 = local write "new picture"(w938) -> ()
                  }
                  frame True {
                    n391 = One Button Dialog(message="顶升横梁与踏步已连接，请取消下回转支座与塔身连接！" ("消息")) -> ()  [unwired: 1 in, 1 out]
                    n392 = call <vilib>:"Read PNG File.vi"("path to PNG file"=path "Picture_Data/1.png" ("path to JPEG file")) -> ("image data"=w942:T5)  [unwired: 8 in, 2 out]
                    n393 = local write "操作规范"("顶升横梁与踏步已连接，请取消下回转支座与塔身连接！" ("字符串")) -> ()
                    n394 = call <vilib>:"Draw Flattened Pixmap.vi"("image data"=w942) -> ("new picture"=w941:picture)  [unwired: 8 in]
                    n395 = local write "new picture"(w941) -> ()
                  }
                }
                n396 = Equal?(x=w749, y=1) -> (x = y?=w751:bool)
                n397 = Equal?(x=w748, y=1) -> (x = y?=w752:bool)
                n398 = Equal?(x=w739, y=1) -> (x = y?=w762:bool)
                n399 = Equal?(x=w738, y=1) -> (x = y?=w763:bool)
                n400 = Equal?(x=w740, y=1) -> (x = y?=w761:bool)
                n401 = Equal?(x=w741, y=1) -> (x = y?=w759:bool)
                n402 = Equal?(x=w747, y=0) -> (x = y?=w753:bool)
                n403 = Equal?(x=w742, y=0) -> (x = y?=w758:bool)
                n404 = Equal?(x=w744, y=0) -> (x = y?=w756:bool)
                n405 = Equal?(x=w745, y=0) -> (x = y?=w755:bool)
                n406 = Equal?(x=w743, y=0) -> (x = y?=w757:bool)
                n407 = Equal?(x=w734, y=1) -> (x = y?=w760:bool)
                n408 = Equal?(x=w746, y=0) -> (x = y?=w754:bool)
                n409 = Compound Arithmetic op=AND ("复合运算")(w751, w752, w753, w754, w755, w756, w757, w758, w759, w760, w761, w762, w763) -> (w737:bool)
                n410 = Equal?(x=w749, y=1) -> (x = y?=w776:bool)
                n411 = Equal?(x=w748, y=1) -> (x = y?=w775:bool)
                n412 = Equal?(x=w739, y=1) -> (x = y?=w765:bool)
                n413 = Equal?(x=w738, y=1) -> (x = y?=w764:bool)
                n414 = Equal?(x=w740, y=1) -> (x = y?=w766:bool)
                n415 = Equal?(x=w741, y=1) -> (x = y?=w768:bool)
                n416 = Equal?(x=w747, y=0) -> (x = y?=w774:bool)
                n417 = Equal?(x=w742, y=1) -> (x = y?=w769:bool)
                n418 = Equal?(x=w744, y=1) -> (x = y?=w771:bool)
                n419 = Equal?(x=w745, y=1) -> (x = y?=w772:bool)
                n420 = Equal?(x=w743, y=1) -> (x = y?=w770:bool)
                n421 = Equal?(x=w734, y=1) -> (x = y?=w767:bool)
                n422 = Equal?(x=w746, y=0) -> (x = y?=w773:bool)
                n423 = Compound Arithmetic op=AND ("复合运算")(w776, w775, w774, w773, w772, w771, w770, w769, w768, w767, w766, w765, w764) -> (w736:bool)
                n424 = Equal?(x=w749, y=0) -> (x = y?=w777:bool)
                n425 = Equal?(x=w748, y=0) -> (x = y?=w778:bool)
                n426 = Equal?(x=w739, y=1) -> (x = y?=w788:bool)
                n427 = Equal?(x=w738, y=1) -> (x = y?=w789:bool)
                n428 = Equal?(x=w740, y=1) -> (x = y?=w787:bool)
                n429 = Equal?(x=w741, y=1) -> (x = y?=w785:bool)
                n430 = Equal?(x=w747, y=0) -> (x = y?=w779:bool)
                n431 = Equal?(x=w742, y=1) -> (x = y?=w784:bool)
                n432 = Equal?(x=w744, y=1) -> (x = y?=w782:bool)
                n433 = Equal?(x=w745, y=1) -> (x = y?=w781:bool)
                n434 = Equal?(x=w743, y=1) -> (x = y?=w783:bool)
                n435 = Equal?(x=w734, y=1) -> (x = y?=w786:bool)
                n436 = Equal?(x=w746, y=0) -> (x = y?=w780:bool)
                n437 = Compound Arithmetic op=AND ("复合运算")(w777, w778, w779, w780, w781, w782, w783, w784, w785, w786, w787, w788, w789) -> (w735:bool)
                n438 = case shown="真" w735 {
                  frame False {
                    n439 = call "Empty Picture"() -> ("empty picture"=w909:picture)
                    n440 = local write "new picture"(w909) -> ()
                    n441 = local write "操作规范"("" ("字符串")) -> ()
                  }
                  frame True {
                    n442 = call <vilib>:"Read PNG File.vi"("path to PNG file"=path "Picture_Data/1.png" ("path to JPEG file")) -> ("image data"=w915:T5)  [unwired: 8 in, 2 out]
                    n443 = call <vilib>:"Draw Flattened Pixmap.vi"("image data"=w915) -> ("new picture"=w911:picture)  [unwired: 8 in]
                    n444 = One Button Dialog(message="顶升横梁与踏步连接销轴已拆除，请压缩油缸！" ("消息")) -> ()  [unwired: 1 in, 1 out]
                    n445 = local write "new picture"(w911) -> ()
                    n446 = local write "操作规范"("顶升横梁与踏步连接销轴已拆除，请压缩油缸！" ("字符串")) -> ()
                  }
                }
                n447 = case shown="真" w737 {
                  frame False {
                    n448 = call "Empty Picture"() -> ("empty picture"=w923:picture)
                    n449 = local write "new picture"(w923) -> ()
                    n450 = local write "操作规范"("" ("字符串")) -> ()
                  }
                  frame True {
                    n451 = call <vilib>:"Read PNG File.vi"("path to PNG file"=path "Picture_Data/1.png" ("path to JPEG file")) -> ("image data"=w929:T5)  [unwired: 8 in, 2 out]
                    n452 = call <vilib>:"Draw Flattened Pixmap.vi"("image data"=w929) -> ("new picture"=w925:picture)  [unwired: 8 in]
                    n453 = One Button Dialog(message="油缸已就位，请连接下回转支座与塔身！" ("消息")) -> ()  [unwired: 1 in, 1 out]
                    n454 = local write "new picture"(w925) -> ()
                    n455 = local write "操作规范"("油缸已就位，请连接下回转支座与塔身！" ("字符串")) -> ()
                  }
                }
                n456 = case shown="真" w736 {
                  frame False {
                    n457 = call "Empty Picture"() -> ("empty picture"=w916:picture)
                    n458 = local write "new picture"(w916) -> ()
                    n459 = local write "操作规范"("" ("字符串")) -> ()
                  }
                  frame True {
                    n460 = call <vilib>:"Read PNG File.vi"("path to PNG file"=path "Picture_Data/1.png" ("path to JPEG file")) -> ("image data"=w922:T5)  [unwired: 8 in, 2 out]
                    n461 = call <vilib>:"Draw Flattened Pixmap.vi"("image data"=w922) -> ("new picture"=w918:picture)  [unwired: 8 in]
                    n462 = One Button Dialog(message="下回转与塔身已连接，请拆除顶升横梁与踏步连接销轴！" ("消息")) -> ()  [unwired: 1 in, 1 out]
                    n463 = local write "new picture"(w918) -> ()
                    n464 = local write "操作规范"("下回转与塔身已连接，请拆除顶升横梁与踏步连接销轴！" ("字符串")) -> ()
                  }
                }
              }
              frame 158..168 {
                n465 = Equal?(x=w964, y=1) -> (x = y?=w1017:bool)
                n466 = Equal?(x=w965, y=1) -> (x = y?=w1016:bool)
                n467 = Equal?(x=w954, y=0) -> (x = y?=w1006:bool)
                n468 = Equal?(x=w953, y=0) -> (x = y?=w1005:bool)
                n469 = Equal?(x=w955, y=0) -> (x = y?=w1007:bool)
                n470 = Equal?(x=w957, y=0) -> (x = y?=w1009:bool)
                n471 = Equal?(x=w963, y=0) -> (x = y?=w1015:bool)
                n472 = Equal?(x=w958, y=0) -> (x = y?=w1010:bool)
                n473 = Equal?(x=w960, y=0) -> (x = y?=w1012:bool)
                n474 = Equal?(x=w961, y=0) -> (x = y?=w1013:bool)
                n475 = Equal?(x=w959, y=0) -> (x = y?=w1011:bool)
                n476 = Equal?(x=w956, y=0) -> (x = y?=w1008:bool)
                n477 = Equal?(x=w962, y=0) -> (x = y?=w1014:bool)
                n478 = Compound Arithmetic op=AND ("复合运算")(w1017, w1016, w1015, w1014, w1013, w1012, w1011, w1010, w1009, w1008, w1007, w1006, w1005) -> (w952:bool)
                n479 = Equal?(x=w964, y=1) -> (x = y?=w992:bool)
                n480 = Equal?(x=w965, y=1) -> (x = y?=w993:bool)
                n481 = Equal?(x=w954, y=0) -> (x = y?=w1003:bool)
                n482 = Equal?(x=w953, y=0) -> (x = y?=w1004:bool)
                n483 = Equal?(x=w955, y=0) -> (x = y?=w1002:bool)
                n484 = Equal?(x=w957, y=0) -> (x = y?=w1000:bool)
                n485 = Equal?(x=w963, y=1) -> (x = y?=w994:bool)
                n486 = Equal?(x=w958, y=0) -> (x = y?=w999:bool)
                n487 = Equal?(x=w960, y=0) -> (x = y?=w997:bool)
                n488 = Equal?(x=w961, y=0) -> (x = y?=w996:bool)
                n489 = Equal?(x=w959, y=0) -> (x = y?=w998:bool)
                n490 = Equal?(x=w956, y=0) -> (x = y?=w1001:bool)
                n491 = Equal?(x=w962, y=1) -> (x = y?=w995:bool)
                n492 = Compound Arithmetic op=AND ("复合运算")(w992, w993, w994, w995, w996, w997, w998, w999, w1000, w1001, w1002, w1003, w1004) -> (w951:bool)
                n493 = case shown="真" w952 {
                  frame False {
                    (unwired) "" ("字符串")
                    n494 = call "Empty Picture"() -> ()  [unwired: 1 out]
                  }
                  frame True {
                    n495 = call <vilib>:"Read PNG File.vi"("path to PNG file"=path "Picture_Data/1.png" ("path to JPEG file")) -> ("image data"=w1027:T5)  [unwired: 8 in, 2 out]
                    n496 = local write "操作规范"("顶升油缸已到位，请压下爬爪！" ("字符串")) -> ()
                    n497 = call <vilib>:"Draw Flattened Pixmap.vi"("image data"=w1027) -> ("new picture"=w1023:picture)  [unwired: 8 in]
                    n498 = One Button Dialog(message="顶升油缸已到位，请压下爬爪！" ("消息")) -> ()  [unwired: 1 in, 1 out]
                    n499 = local write "new picture"(w1023) -> ()
                  }
                }
                n500 = case shown="真" w951 {
                  frame False {
                    (unwired) "" ("字符串")
                    n501 = call "Empty Picture"() -> ()  [unwired: 1 out]
                  }
                  frame True {
                    n502 = call <vilib>:"Read PNG File.vi"("path to PNG file"=path "Picture_Data/1.png" ("path to JPEG file")) -> ("image data"=w1022:T5)  [unwired: 8 in, 2 out]
                    n503 = local write "操作规范"("爬爪已就位，请压缩油缸！" ("字符串")) -> ()
                    n504 = call <vilib>:"Draw Flattened Pixmap.vi"("image data"=w1022) -> ("new picture"=w1018:picture)  [unwired: 8 in]
                    n505 = One Button Dialog(message="爬爪已就位，请压缩油缸！" ("消息")) -> ()  [unwired: 1 in, 1 out]
                    n506 = local write "new picture"(w1018) -> ()
                  }
                }
              }
              frame 150..155 {
                n507 = Equal?(x=w1042, y=1) -> (x = y?=w1094:bool)
                n508 = Equal?(x=w1041, y=1) -> (x = y?=w1093:bool)
                n509 = Equal?(x=w1031, y=0) -> (x = y?=w1083:bool)
                n510 = Equal?(x=w1030, y=0) -> (x = y?=w1082:bool)
                n511 = Equal?(x=w1032, y=0) -> (x = y?=w1084:bool)
                n512 = Equal?(x=w1034, y=0) -> (x = y?=w1086:bool)
                n513 = Equal?(x=w1040, y=1) -> (x = y?=w1092:bool)
                n514 = Equal?(x=w1035, y=0) -> (x = y?=w1087:bool)
                n515 = Equal?(x=w1037, y=0) -> (x = y?=w1089:bool)
                n516 = Equal?(x=w1038, y=0) -> (x = y?=w1090:bool)
                n517 = Equal?(x=w1036, y=0) -> (x = y?=w1088:bool)
                n518 = Equal?(x=w1033, y=0) -> (x = y?=w1085:bool)
                n519 = Equal?(x=w1039, y=1) -> (x = y?=w1091:bool)
                n520 = Compound Arithmetic op=AND ("复合运算")(w1094, w1093, w1092, w1091, w1090, w1089, w1088, w1087, w1086, w1085, w1084, w1083, w1082) -> (w1029:bool)
                n521 = Equal?(x=w1042, y=0) -> (x = y?=w1069:bool)
                n522 = Equal?(x=w1041, y=0) -> (x = y?=w1070:bool)
                n523 = Equal?(x=w1031, y=0) -> (x = y?=w1080:bool)
                n524 = Equal?(x=w1030, y=0) -> (x = y?=w1081:bool)
                n525 = Equal?(x=w1032, y=0) -> (x = y?=w1079:bool)
                n526 = Equal?(x=w1034, y=0) -> (x = y?=w1077:bool)
                n527 = Equal?(x=w1040, y=1) -> (x = y?=w1071:bool)
                n528 = Equal?(x=w1035, y=0) -> (x = y?=w1076:bool)
                n529 = Equal?(x=w1037, y=0) -> (x = y?=w1074:bool)
                n530 = Equal?(x=w1038, y=0) -> (x = y?=w1073:bool)
                n531 = Equal?(x=w1036, y=0) -> (x = y?=w1075:bool)
                n532 = Equal?(x=w1033, y=0) -> (x = y?=w1078:bool)
                n533 = Equal?(x=w1039, y=1) -> (x = y?=w1072:bool)
                n534 = Compound Arithmetic op=AND ("复合运算")(w1069, w1070, w1071, w1072, w1073, w1074, w1075, w1076, w1077, w1078, w1079, w1080, w1081) -> (w1028:bool)
                n535 = case shown="真" w1028 {
                  frame False {
                    (unwired) "" ("字符串")
                    n536 = call "Empty Picture"() -> ()  [unwired: 1 out]
                  }
                  frame True {
                    n537 = call <vilib>:"Read PNG File.vi"("path to PNG file"=path "Picture_Data/1.png" ("path to JPEG file")) -> ("image data"=w1099:T5)  [unwired: 8 in, 2 out]
                    n538 = call <vilib>:"Draw Flattened Pixmap.vi"("image data"=w1099) -> ("new picture"=w1095:picture)  [unwired: 8 in]
                    n539 = One Button Dialog(message="顶升横梁与踏步连接销轴已拆除，请压缩油缸！" ("消息")) -> ()  [unwired: 1 in, 1 out]
                    n540 = local write "操作规范"("顶升横梁与踏步连接销轴已拆除，请压缩油缸！" ("字符串")) -> ()
                    n541 = local write "new picture"(w1095) -> ()
                  }
                }
                n542 = case shown="真" w1029 {
                  frame False {
                    (unwired) "" ("字符串")
                    n543 = call "Empty Picture"() -> ()  [unwired: 1 out]
                  }
                  frame True {
                    n544 = call <vilib>:"Read PNG File.vi"("path to PNG file"=path "Picture_Data/1.png" ("path to JPEG file")) -> ("image data"=w1104:T5)  [unwired: 8 in, 2 out]
                    n545 = call <vilib>:"Draw Flattened Pixmap.vi"("image data"=w1104) -> ("new picture"=w1100:picture)  [unwired: 8 in]
                    n546 = One Button Dialog(message="油缸已回缩就位，请拆除顶升横梁与踏步连接销轴！" ("消息")) -> ()  [unwired: 1 in, 1 out]
                    n547 = local write "操作规范"("油缸已回缩就位，请拆除顶升横梁与踏步连接销轴！" ("字符串")) -> ()
                    n548 = local write "new picture"(w1100) -> ()
                  }
                }
              }
              frame 120..130 {
                n549 = Equal?(x=w1117, y=1) -> (x = y?=w1171:bool)
                n550 = Equal?(x=w1116, y=1) -> (x = y?=w1170:bool)
                n551 = Equal?(x=w1106, y=0) -> (x = y?=w1160:bool)
                n552 = Equal?(x=w1105, y=0) -> (x = y?=w1159:bool)
                n553 = Equal?(x=w1107, y=0) -> (x = y?=w1161:bool)
                n554 = Equal?(x=w1109, y=0) -> (x = y?=w1163:bool)
                n555 = Equal?(x=w1115, y=0) -> (x = y?=w1169:bool)
                n556 = Equal?(x=w1110, y=0) -> (x = y?=w1164:bool)
                n557 = Equal?(x=w1112, y=0) -> (x = y?=w1166:bool)
                n558 = Equal?(x=w1113, y=0) -> (x = y?=w1167:bool)
                n559 = Equal?(x=w1111, y=0) -> (x = y?=w1165:bool)
                n560 = Equal?(x=w1108, y=0) -> (x = y?=w1162:bool)
                n561 = Equal?(x=w1114, y=0) -> (x = y?=w1168:bool)
                n562 = Compound Arithmetic op=AND ("复合运算")(w1171, w1170, w1169, w1168, w1167, w1166, w1165, w1164, w1163, w1162, w1161, w1160, w1159) -> (w1119:bool)
                n563 = Equal?(x=w1117, y=1) -> (x = y?=w1146:bool)
                n564 = Equal?(x=w1116, y=1) -> (x = y?=w1147:bool)
                n565 = Equal?(x=w1106, y=0) -> (x = y?=w1157:bool)
                n566 = Equal?(x=w1105, y=1) -> (x = y?=w1158:bool)
                n567 = Equal?(x=w1107, y=0) -> (x = y?=w1156:bool)
                n568 = Equal?(x=w1109, y=0) -> (x = y?=w1154:bool)
                n569 = Equal?(x=w1115, y=0) -> (x = y?=w1148:bool)
                n570 = Equal?(x=w1110, y=0) -> (x = y?=w1153:bool)
                n571 = Equal?(x=w1112, y=0) -> (x = y?=w1151:bool)
                n572 = Equal?(x=w1113, y=0) -> (x = y?=w1150:bool)
                n573 = Equal?(x=w1111, y=0) -> (x = y?=w1152:bool)
                n574 = Equal?(x=w1108, y=0) -> (x = y?=w1155:bool)
                n575 = Equal?(x=w1114, y=0) -> (x = y?=w1149:bool)
                n576 = Compound Arithmetic op=AND ("复合运算")(w1146, w1147, w1148, w1149, w1150, w1151, w1152, w1153, w1154, w1155, w1156, w1157, w1158) -> (w1118:bool)
                n577 = case shown="真" w1119 {
                  frame False {
                    n578 = call "Empty Picture"() -> ("empty picture"=w1180:picture)
                    n579 = local write "操作规范"("" ("字符串")) -> ()
                    n580 = local write "new picture"(w1180) -> ()
                  }
                  frame True {
                    n581 = call <vilib>:"Read PNG File.vi"("path to PNG file"=path "Picture_Data/1.png" ("path to JPEG file")) -> ("image data"=w1185:T5)  [unwired: 8 in, 2 out]
                    n582 = call <vilib>:"Draw Flattened Pixmap.vi"("image data"=w1185) -> ("new picture"=w1181:picture)  [unwired: 8 in]
                    n583 = One Button Dialog(message="顶升油缸已就位，请引进新标准节！" ("消息")) -> ()  [unwired: 1 in, 1 out]
                    n584 = local write "操作规范"("顶升油缸已就位，请引进新标准节！" ("字符串")) -> ()
                    n585 = local write "new picture"(w1181) -> ()
                  }
                }
                n586 = case shown="真" w1118 {
                  frame False {
                    n587 = call "Empty Picture"() -> ("empty picture"=w1172:picture)
                    n588 = local write "new picture"(w1172) -> ()
                    n589 = local write "操作规范"("" ("字符串")) -> ()
                  }
                  frame True {
                    n590 = call <vilib>:"Read PNG File.vi"("path to PNG file"=path "Picture_Data/1.png" ("path to JPEG file")) -> ("image data"=w1178:T5)  [unwired: 8 in, 2 out]
                    n591 = call <vilib>:"Draw Flattened Pixmap.vi"("image data"=w1178) -> ("new picture"=w1174:picture)  [unwired: 8 in]
                    n592 = One Button Dialog(message="新标准节已引进，请压缩油缸！" ("消息")) -> ()  [unwired: 1 in, 1 out]
                    n593 = local write "操作规范"("新标准节已引进，请压缩油缸！" ("字符串")) -> ()
                    n594 = local write "new picture"(w1174) -> ()
                  }
                }
              }
              frame 170..180 {
                n595 = One Button Dialog(message="顶升冒顶警告！" ("消息")) -> ()  [unwired: 1 in, 1 out]
              }
              frame 110..115 {
                n596 = Equal?(x=w1199, y=1) -> (x = y?=w1226:bool)
                n597 = Equal?(x=w1198, y=1) -> (x = y?=w1227:bool)
                n598 = Equal?(x=w1188, y=0) -> (x = y?=w1237:bool)
                n599 = Equal?(x=w1187, y=1) -> (x = y?=w1238:bool)
                n600 = Equal?(x=w1189, y=0) -> (x = y?=w1236:bool)
                n601 = Equal?(x=w1191, y=0) -> (x = y?=w1234:bool)
                n602 = Equal?(x=w1197, y=0) -> (x = y?=w1228:bool)
                n603 = Equal?(x=w1192, y=0) -> (x = y?=w1233:bool)
                n604 = Equal?(x=w1194, y=0) -> (x = y?=w1231:bool)
                n605 = Equal?(x=w1195, y=0) -> (x = y?=w1230:bool)
                n606 = Equal?(x=w1193, y=0) -> (x = y?=w1232:bool)
                n607 = Equal?(x=w1190, y=0) -> (x = y?=w1235:bool)
                n608 = Equal?(x=w1196, y=0) -> (x = y?=w1229:bool)
                n609 = Compound Arithmetic op=AND ("复合运算")(w1226, w1227, w1228, w1229, w1230, w1231, w1232, w1233, w1234, w1235, w1236, w1237, w1238) -> (w1252:bool)
                n610 = Equal?(x=w1199, y=1) -> (x = y?=w1251:bool)
                n611 = Equal?(x=w1198, y=1) -> (x = y?=w1250:bool)
                n612 = Equal?(x=w1188, y=1) -> (x = y?=w1240:bool)
                n613 = Equal?(x=w1187, y=1) -> (x = y?=w1239:bool)
                n614 = Equal?(x=w1189, y=1) -> (x = y?=w1241:bool)
                n615 = Equal?(x=w1191, y=1) -> (x = y?=w1243:bool)
                n616 = Equal?(x=w1197, y=0) -> (x = y?=w1249:bool)
                n617 = Equal?(x=w1192, y=0) -> (x = y?=w1244:bool)
                n618 = Equal?(x=w1194, y=0) -> (x = y?=w1246:bool)
                n619 = Equal?(x=w1195, y=0) -> (x = y?=w1247:bool)
                n620 = Equal?(x=w1193, y=0) -> (x = y?=w1245:bool)
                n621 = Equal?(x=w1190, y=1) -> (x = y?=w1242:bool)
                n622 = Equal?(x=w1196, y=0) -> (x = y?=w1248:bool)
                n623 = Compound Arithmetic op=AND ("复合运算")(w1251, w1250, w1249, w1248, w1247, w1246, w1245, w1244, w1243, w1242, w1241, w1240, w1239) -> (w1253:bool)
                n624 = case shown="真" w1253 {
                  frame False {
                    n625 = call "Empty Picture"() -> ("empty picture"=w1254:picture)
                    n626 = local write "new picture"(w1254) -> ()
                    n627 = local write "操作规范"("" ("字符串")) -> ()
                  }
                  frame True {
                    n628 = call <vilib>:"Read PNG File.vi"("path to PNG file"=path "Picture_Data/1.png" ("path to JPEG file")) -> ("image data"=w1260:T5)  [unwired: 8 in, 2 out]
                    n629 = call <vilib>:"Draw Flattened Pixmap.vi"("image data"=w1260) -> ("new picture"=w1256:picture)  [unwired: 8 in]
                    n630 = One Button Dialog(message="标准节与塔身已连接，请压缩油缸！" ("消息")) -> ()  [unwired: 1 in, 1 out]
                    n631 = local write "new picture"(w1256) -> ()
                    n632 = local write "操作规范"("标准节与塔身已连接，请压缩油缸！" ("字符串")) -> ()
                  }
                }
                n633 = case shown="真" w1252 {
                  frame False {
                    n634 = call "Empty Picture"() -> ("empty picture"=w1261:picture)
                    n635 = local write "new picture"(w1261) -> ()
                    n636 = local write "操作规范"("" ("字符串")) -> ()
                  }
                  frame True {
                    n637 = call <vilib>:"Read PNG File.vi"("path to PNG file"=path "Picture_Data/1.png" ("path to JPEG file")) -> ("image data"=w1267:T5)  [unwired: 8 in, 2 out]
                    n638 = call <vilib>:"Draw Flattened Pixmap.vi"("image data"=w1267) -> ("new picture"=w1263:picture)  [unwired: 8 in]
                    n639 = One Button Dialog(message="油缸已就位，请连接引进节与塔身！" ("消息")) -> ()  [unwired: 1 in, 1 out]
                    n640 = local write "new picture"(w1263) -> ()
                    n641 = local write "操作规范"("油缸已就位，请连接引进节与塔身！" ("字符串")) -> ()
                  }
                }
              }
            }
            "data out" <- w593
          }
        }
        n642 = property on="数据输出" class="Str"("Text.Scroll Position"=inf) -> ()  [unwired: 2 in, 2 out]
      }
    }
    n643 = String Length(string=w54) -> (length=w89:i32)
    n644 = Not Equal To 0?(x=w89) -> (x != 0?=w88:bool)
    n645 = case shown="真" w88 {
      tunnel: w54 -> [_ w453]
      frame False {
      }
      frame True {
        n646 = local read "开始配平"() -> (w454:bool)
        n647 = local read "数据输出 2"() -> (w452:string)
        n648 = case shown="真" w454 {
          tunnel: w453 -> [_ w482]
          tunnel: w452 -> [_ w485]
          frame False {
          }
          frame True {
            n649 = Concatenate Strings(w485, "\n", w482) -> (→"数据输出 2":string)
            n650 = String Subset(string=w482, offset (0)=1 ("偏移量(0)"), length (rest)=3 ("长度（剩余）")) -> (substring=w473:string)
            "子字符串" <- w473
            n651 = String Subset(string=w482, offset (0)=11 ("偏移量(0)"), length (rest)=3 ("长度（剩余）")) -> (substring=w469:string)
            "子字符串 3" <- w469
            n652 = String Subset(string=w482, offset (0)=16 ("偏移量(0)"), length (rest)=3 ("长度（剩余）")) -> (substring=w467:string)
            "子字符串 4" <- w467
            n653 = String Subset(string=w482, offset (0)=6 ("偏移量(0)"), length (rest)=3 ("长度（剩余）")) -> (substring=w470:string)
            "子字符串 2" <- w470
            n654 = Fract/Exp String To Number(string=w473, offset=0 ("偏移量")) -> (number=w465:dbl)  [unwired: 2 in, 1 out]
            "超声波雷达1" <- w465
            "超声波雷达1" <- w465
            n655 = Fract/Exp String To Number(string=w470, offset=0 ("默认(0 I32)")) -> (number=w464:dbl)  [unwired: 2 in, 1 out]
            "超声波雷达2" <- w464
            "超声波雷达2" <- w464
            n656 = Fract/Exp String To Number(string=w469, offset=0 ("默认(0 I32)")) -> (number=w456:dbl)  [unwired: 2 in, 1 out]
            "?" <- w456
            "超声波雷达35" <- w456
            n657 = Fract/Exp String To Number(string=w467, offset=0 ("偏移量")) -> (number=w455:dbl)  [unwired: 2 in, 1 out]
            "超声波雷达4 6" <- w455
            "超声波雷达4" <- w455
            n658 = Subtract(x=w456, y=w455) -> (x-y=w457:dbl)
            n659 = Subtract(x=w465, y=w464) -> (x-y=w463:dbl)
            n660 = Absolute Value(x=w457) -> (abs(x)=w458:dbl)
            n661 = Absolute Value(x=w463) -> (abs(x)=w462:dbl)
            n662 = Less?(x=w458, y=10.0) -> ()  [unwired: 1 out]
            n663 = Less?(x=w462, y=10.0) -> (x < y?=→"配平指示1":bool)
          }
        }
        n664 = property on="数据输出" class="Str"("Text.Scroll Position"=inf) -> ()  [unwired: 2 in, 2 out]
      }
    }
    n665 = case shown="真" "清空" {
      frame False {
      }
      frame True {
        n666 = local write "数据输出"("" ("数据输出")) -> ()
      }
    }
    n667 = case shown="真" "清空 2" {
      frame False {
      }
      frame True {
        n668 = local write "数据输出 2"("" ("数据输出")) -> ()
      }
    }
    n669 = Greater Or Equal?(x=w48, y=5.0) -> (x >= y?=w47:bool)
    n670 = Greater Or Equal?(x=w46, y=5.0) -> (x >= y?=w45:bool)
    n671 = case shown="真" w47 {
      frame False {
      }
      frame True {
        n672 = call <vilib>:"Read PNG File.vi"("path to PNG file"=path "Picture_Data/1.png" ("path to JPEG file")) -> ("image data"=w208:T5)  [unwired: 8 in, 2 out]
        n673 = call <vilib>:"Draw Flattened Pixmap.vi"("image data"=w208) -> ("new picture"=→"new picture 2":picture)  [unwired: 8 in]
        n674 = One Button Dialog(message="警告！顶升套架y轴倾角过大，请立即停止升降节！" ("消息")) -> ()  [unwired: 1 in, 1 out]
      }
    }
    n675 = Greater Or Equal?(x=w42, y=3.0) -> (x >= y?=w40:bool)
    n676 = case shown="真" w40 {
      frame False {
      }
      frame True {
        n677 = call <vilib>:"Read PNG File.vi"("path to PNG file"=path "Picture_Data/1.png" ("path to JPEG file")) -> ("image data"=w200:T5)  [unwired: 8 in, 2 out]
        n678 = call <vilib>:"Draw Flattened Pixmap.vi"("image data"=w200) -> ("new picture"=→"new picture 4":picture)  [unwired: 8 in]
        n679 = One Button Dialog(message="警告！风速过大，请立即停止升降节！" ("消息")) -> ()  [unwired: 1 in, 1 out]
      }
    }
    n680 = case shown="真" w45 {
      frame False {
      }
      frame True {
        n681 = call <vilib>:"Read PNG File.vi"("path to PNG file"=path "Picture_Data/1.png" ("path to JPEG file")) -> ("image data"=w204:T5)  [unwired: 8 in, 2 out]
        n682 = call <vilib>:"Draw Flattened Pixmap.vi"("image data"=w204) -> ("new picture"=→"new picture 3":picture)  [unwired: 8 in]
        n683 = One Button Dialog(message="警告！顶升套架x轴倾角过大，请立即停止升降节！" ("消息")) -> ()  [unwired: 1 in, 1 out]
      }
    }
    n684 = Number To Fractional String(number=w48) -> (F-format string=w62:string)  [unwired: 3 in]
    n685 = Number To Fractional String(number=w46) -> (F-format string=w63:string)  [unwired: 3 in]
    n686 = Number To Fractional String(number=w42) -> (F-format string=w68:string)  [unwired: 3 in]
    n687 = Number To Fractional String(number=w72) -> (F-format string=w71:string)  [unwired: 3 in]
    n688 = Number To Fractional String(number=w65) -> (F-format string=w61:string)  [unwired: 3 in]
    n689 = Number To Fractional String(number=w64) -> (F-format string=w58:string)  [unwired: 3 in]
    n690 = call <vilib>:"Read PNG File.vi"("path to PNG file"=path "Picture_Data/jacking_beam.png" ("path to JPEG file")) -> ("image data"=w128:T5)  [unwired: 8 in, 2 out]
    n691 = call <vilib>:"Read PNG File.vi"("path to PNG file"=path "Picture_Data/stanard_section.png" ("path to JPEG file")) -> ("image data"=w50:T5)  [unwired: 8 in, 2 out]
    n692 = call <vilib>:"Read PNG File.vi"("path to PNG file"=path "Picture_Data/pin_shaft.png" ("path to JPEG file")) -> ("image data"=w123:T5)  [unwired: 8 in, 2 out]
    n693 = call <vilib>:"Draw Flattened Pixmap.vi"("image data"=w128) -> ("new picture"=→"jacking_beam":picture)  [unwired: 8 in]
    n694 = call <vilib>:"Draw Flattened Pixmap.vi"("image data"=w50) -> ("new picture"=→"stanard_section 2":picture)  [unwired: 8 in]
    n695 = call <vilib>:"Draw Flattened Pixmap.vi"("image data"=w123) -> ("new picture"=→"pin_shaft":picture)  [unwired: 8 in]
    n696 = Concatenate Strings("Device_ID:001,Jacking_frame_x_axis:", "lack_usb" ("字符串"), ",Jacking_frame_y_axis:" ("字符串"), "lack_usb" ("字符串"), ",Jacking_height:" ("字符串"), w71, ",Wind_Speed:" ("字符串"), w68, ",Tower_Crane_body_x_axis:" ("字符串"), w63, ",Tower_Crane_body_y_axis:" ("字符串"), w62, ",Amplitude_Length:" ("字符串"), w61, ",Rotation_Angle:" ("字符串"), w58, ",Photoelectric_Switch:" ("字符串"), w55, ",Radar:" ("字符串"), w54) -> (w77:string)
    n697 = UDP Write(address=w85, port or service name=u16 10000 ("端口或服务名称"), connection ID=w86, data in=w77, 8:w82) -> (error out=w80:errorcluster, 3:w81:refnum<k16>)  [unwired: 1 in]
    n698 = call <vilib>:"Read PNG File.vi"("path to PNG file"=path "Picture_Data/rotary_support.png" ("path to JPEG file")) -> ("image data"=w117:T5)  [unwired: 8 in, 2 out]
    n699 = call <vilib>:"Read PNG File.vi"("path to PNG file"=path "Picture_Data/stanard_section.png" ("path to JPEG file")) -> ("image data"=w122:T5)  [unwired: 8 in, 2 out]
    n700 = call <vilib>:"Draw Flattened Pixmap.vi"("image data"=w117) -> ("new picture"=→"rotary_support":picture)  [unwired: 8 in]
    n701 = call <vilib>:"Draw Flattened Pixmap.vi"("image data"=w122) -> ("new picture"=→"stanard_section":picture)  [unwired: 8 in]
    n702 = call <vilib>:"Read PNG File.vi"("path to PNG file"=path "Picture_Data/section_connect.png" ("path to JPEG file")) -> ("image data"=w114:T5)  [unwired: 8 in, 2 out]
    n703 = call <vilib>:"Draw Flattened Pixmap.vi"("image data"=w114) -> ("new picture"=→"section_connect":picture)  [unwired: 8 in]
  }
  n704 = call <vilib>:"IMAQdx Open Camera.vi"("error in"="error in", "Session In"=T2 "cam0") -> ("error out"=w23:errorcluster, "Session Out"=w24:T2)  [unwired: 8 in]
  n705 = call <vilib>:"IMAQdx Configure Acquisition.vi"("error in"=w23, "Number of Buffers"=u32 3, "Continuous?"=IMAQdx_Acquisition_Mode."Continuous", "Session In"=w24) -> ("error out"=w21:errorcluster, "Session Out"=w22:T2)  [unwired: 6 in]
  n706 = call "IMAQ Create"("Image Name"="test") -> ("New Image"=w11:T1)  [unwired: 4 in, 1 out]
  n707 = call <vilib>:"IMAQdx Start Acquisition.vi"("error in"=w21, "Session In"=w22) -> ("error out"=w19:errorcluster, "Session Out"=w20:T2)  [unwired: 8 in]
  n708 = while {
    shift-right: [w1271] -> w18
    shift-left: w20 -> [w1273]
    shift-right: [w1270] -> w17
    shift-left: w19 -> [w1272]
    shift-right: [w1268] -> w2
    shift-left: w11 -> [w1269]
    stop <- "停止 3" stop-if-true
    n709 = call <vilib>:"IMAQdx Grab2.vi"("error in"=w1272, "Image In"=w1269, "Session In"=w1273) -> ("error out"=w1270:errorcluster, "Image Out"=w1268:T1, "Session Out"=w1271:T2)  [unwired: 5 in, 1 out]
    "视频监控画面1" <- w1268
  }
  n710 = call <vilib>:"IMAQdx Stop Acquisition.vi"("error in"=w17, "Session In"=w18) -> ("error out"=w7:errorcluster, "Session Out"=w4:T2)  [unwired: 8 in]
  n711 = call <vilib>:"IMAQdx Unconfigure Acquisition.vi"("error in"=w7, "Session In"=w4) -> ("error out"=w6:errorcluster, "Session Out"=w3:T2)  [unwired: 8 in]
  n712 = call <vilib>:"IMAQdx Close Camera.vi"("error in"=w6, "Session In"=w3) -> ("error out"=w5:errorcluster)  [unwired: 9 in]
  n713 = call-poly "IMAQ Write File 2"("error in (no error)"=w5, "File Path"="File Path", "Image"=w2) -> ("error out"=w9:errorcluster, "Image Out (duplicate)"=w10:T1)  [unwired: 7 in]
  n714 = call "IMAQ Dispose"("Image"=w10, "error in (no error)"=w9) -> ("error out"=→"error out 2":errorcluster)  [unwired: 4 in]
  n715 = UDP Close(connection ID=w36, 8:w37) -> ()  [unwired: 2 out]
  n716 = UDP Close(connection ID=w26, 8:w25) -> ()  [unwired: 2 out]
  n717 = UDP Close(connection ID=w32, 8:w30) -> ()  [unwired: 2 out]
